vi "Front Panel Control Roll of the Die.vi"() -> ()   [LabVIEW 2019]
uses:
  <vilib>/numeric/Random Number (Range) U64.vi
  <vilib>/numeric/sub_Random U32.vi
panel:
  in  "Press to roll the die":bool
  out "Die shows:":dbl
  # "Challenge: Write a program to roll a die every time you press a button on the front panel."
  # "Try it: Run the program and press the button to roll the die."
  # "You will probably need:\nRandom number generator, Front panel control"
  # "Open the block diagram to see a possible solution."
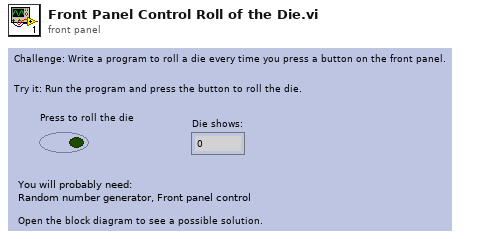
[diagram p1: front panel]
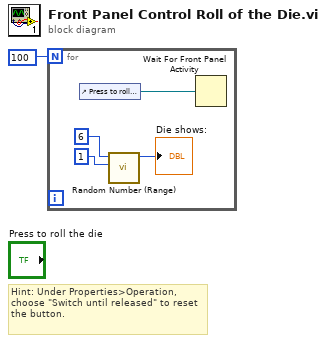
[diagram p0: block diagram]
diagram:
  # "Hint: Under Properties>Operation, choose \"Switch until released\" to reset the button."
  n1 = for {
    N: 100 -> [_]
    n2 = control-ref of="Press to roll the die"() -> (w2:refnum<vi>)
    n3 = call-poly <vilib>:"Random Number (Range).vi"("lower bound (0)"=u64 1, "upper bound (100)"=u64 6) -> ("number"=→"Die shows:":u64)  [unwired: 9 in]
    n4 = Wait For Front Panel Activity(2:w2) -> ()  [unwired: 2 in, 1 out]
  }
